vi "Write dT.vi"(8 "error in (no error)":errorcluster, 10 "dT":dbl, 11 "AcquireTraces in":refnum<class "AcquireTraces.lvclass">) -> (0 "error out":errorcluster, 3 "AcquireTraces out":refnum<class "AcquireTraces.lvclass">)   [LabVIEW 2010, in "AcquireTraces.lvclass"]
uses:
  AcquireTraces.lvclass
  AcquireTraces.lvclass/AcquireTraces.ctl
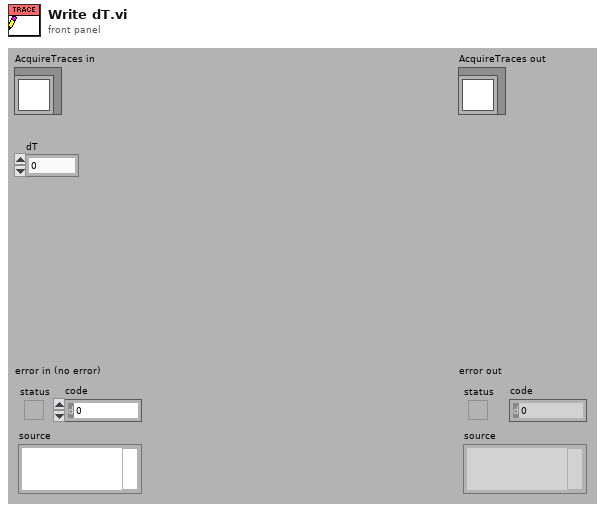
[diagram p1: front panel]
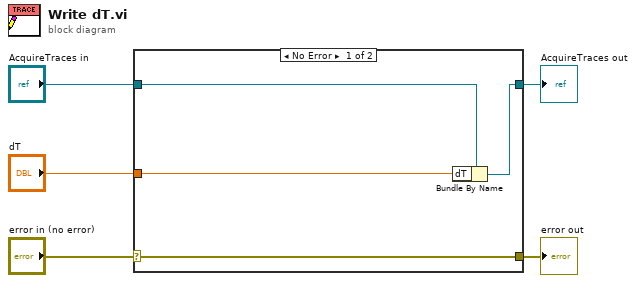
[diagram p0: block diagram]
diagram:
  n1 = case shown="No Error" "error in (no error)" {
    selector: "error in (no error)" -> [w9 w10]
    tunnel: [w9 w10] -> w4
    tunnel: [w7 w11] -> w2
    tunnel: "AcquireTraces in" -> [w8 w11]
    tunnel: "dT" -> [w6 _]
    frame No Error {
      n2 = Bundle By Name(cluster=w8, "dT"=w6) -> (w7:refnum<class "AcquireTraces.lvclass">)
    }
    frame Error {
    }
  }
  "error out" <- w4
  "AcquireTraces out" <- w2
